vi "test.BasicTypes.vi"(8 "error in":errorcluster, 10 "Data":variant, 11 "Command":string) -> (0 "error out":errorcluster, 3 "Return Data":variant)   [LabVIEW 2014]
uses:
  Private/Class/class.GLue.lvclass
  Private/Class/meth.Constructor.vi
  Private/Class/meth.Destructor.vi
  GLue.lvlib
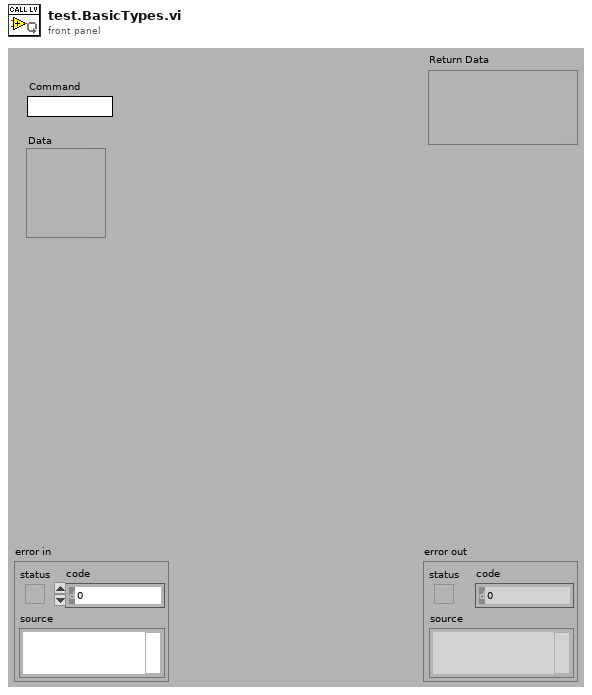
[diagram p1: front panel]
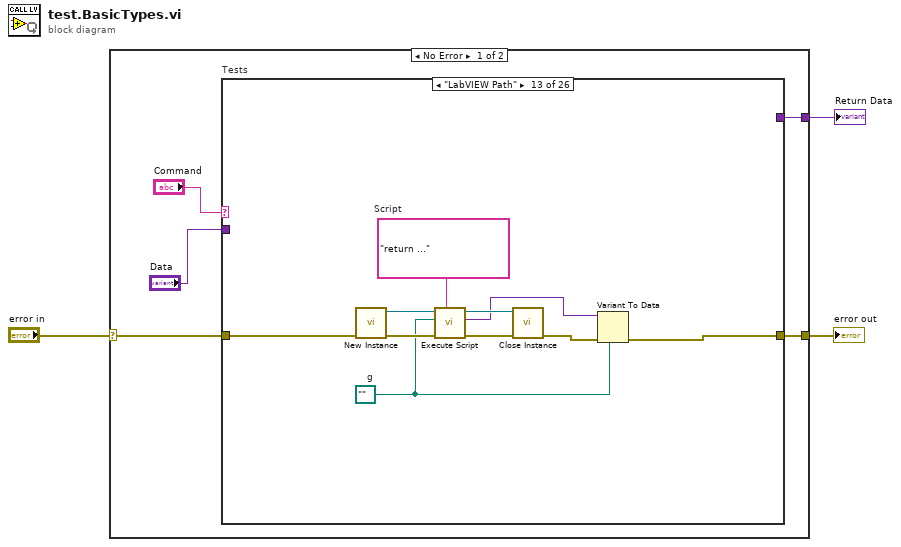
[diagram p0: block diagram]
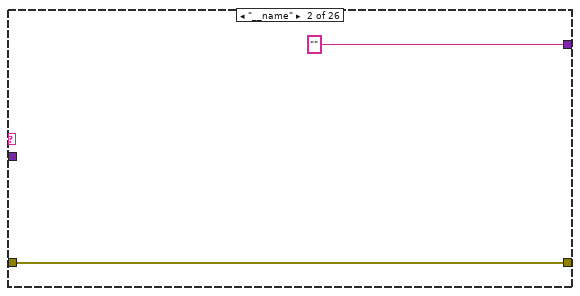
[diagram p3: hidden frame]
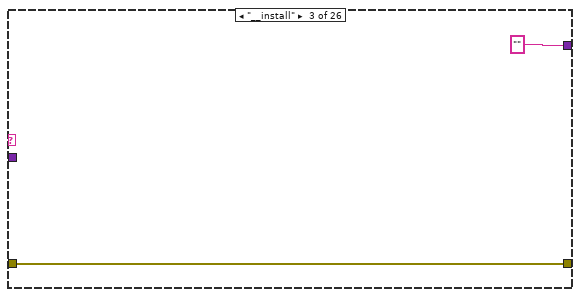
[diagram p4: hidden frame]
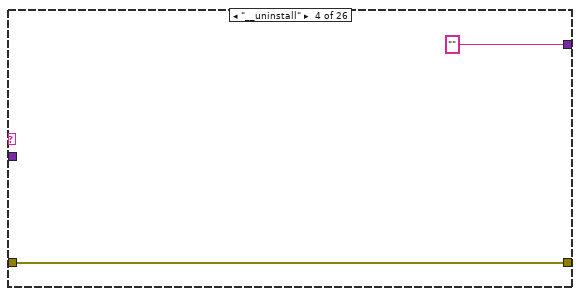
[diagram p5: hidden frame]
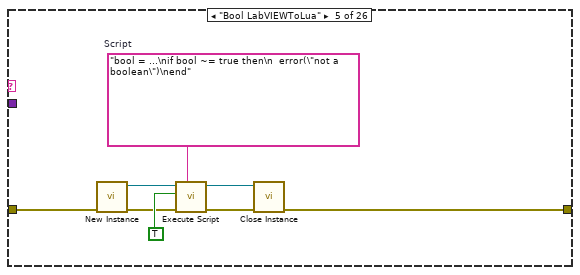
[diagram p6: hidden frame]
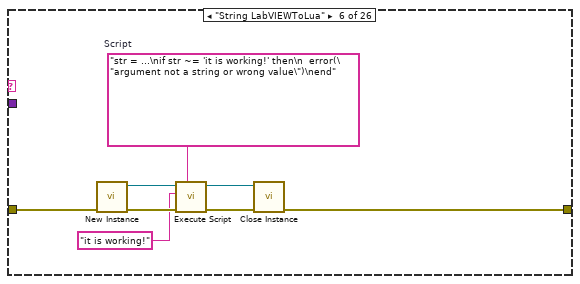
[diagram p7: hidden frame]
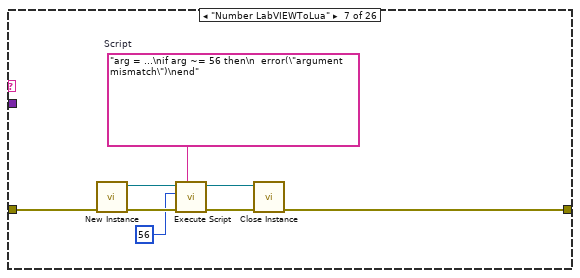
[diagram p8: hidden frame]
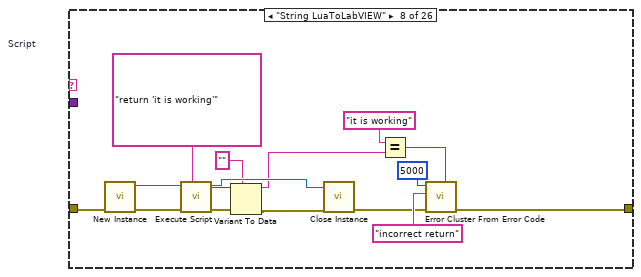
[diagram p9: hidden frame]
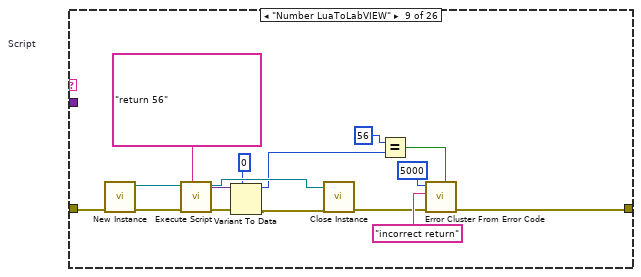
[diagram p10: hidden frame]
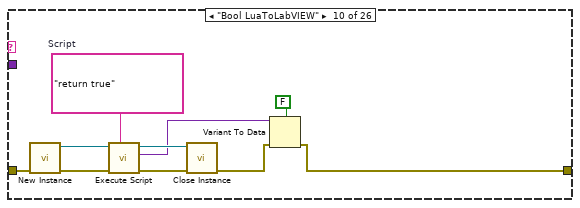
[diagram p11: hidden frame]
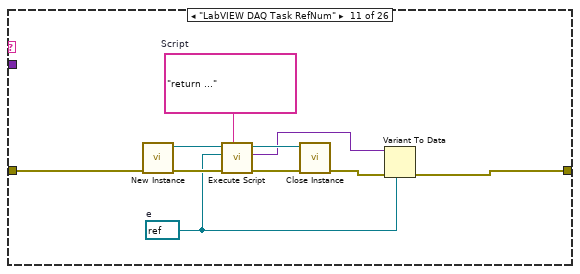
[diagram p12: hidden frame]
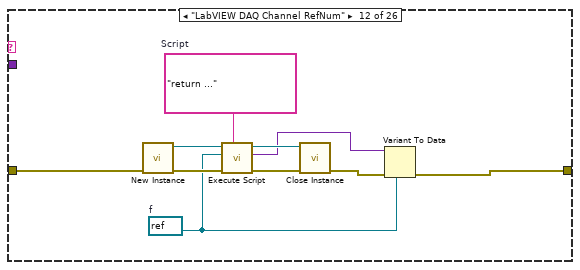
[diagram p13: hidden frame]
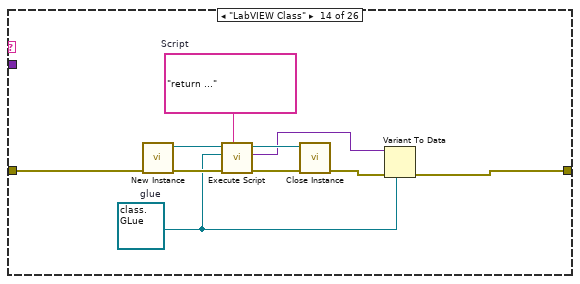
[diagram p14: hidden frame]
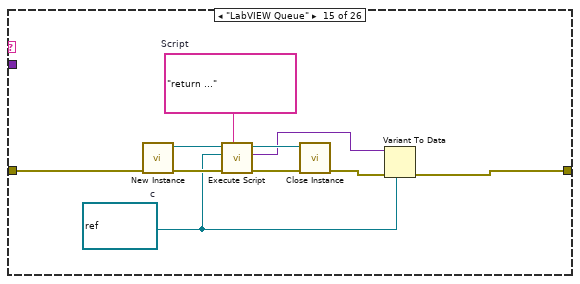
[diagram p15: hidden frame]
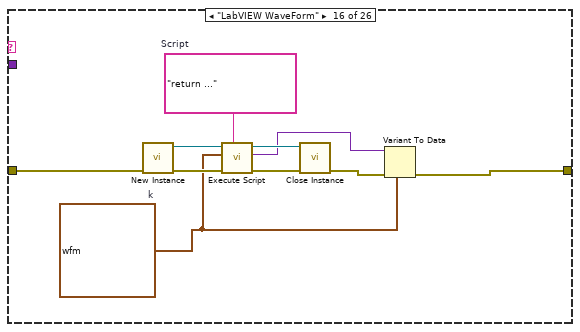
[diagram p16: hidden frame]
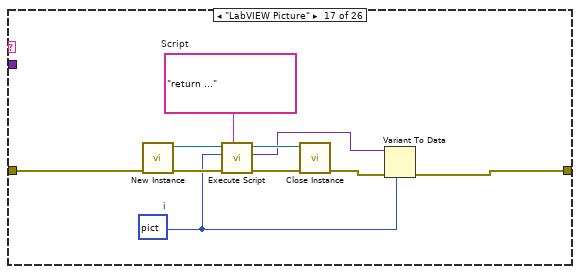
[diagram p17: hidden frame]
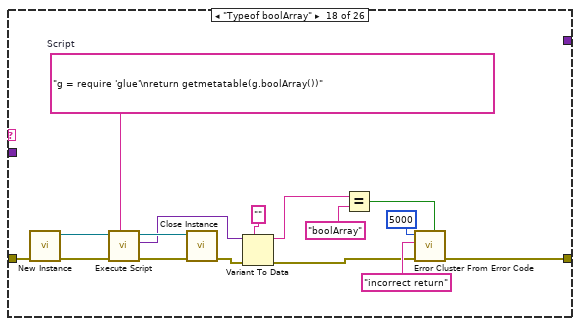
[diagram p18: hidden frame]
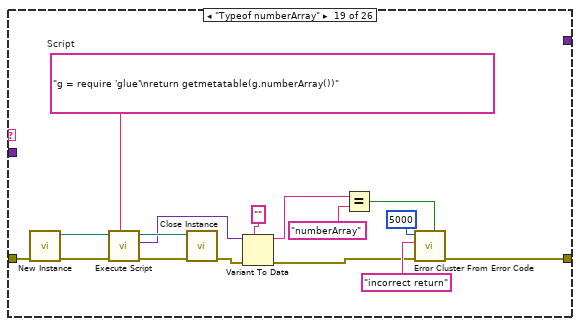
[diagram p19: hidden frame]
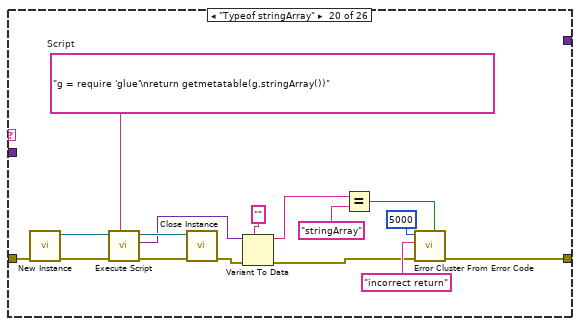
[diagram p20: hidden frame]
diagram:
  n1 = case shown="No Error" "error in" {
    selector: "error in" -> [w8 w297]
    tunnel: [w6 w297] -> w2
    tunnel: [w7 variant ("User Data")] -> w1
    frame No Error {
      n2 = case "Tests" shown="\"LabVIEW Path\"" "Command" {
        tunnel: w8 -> [w10 w11 w13 w15 w18 w27 w35 w53 w69 w77 w87 w97 w107 w117 w127 w137 w147 w163 w179 w195 w211 w227 w243 w260 w275 w290]
        tunnel: "Data" -> [w9 _ _ _ _ _ _ _ _ _ _ _ _ _ _ _ _ _ _ _ _ _ _ _ _ _]
        tunnel: [w9 "" "" "" _ _ _ _ _ _ _ _ _ _ _ _ _ _ _ _ _ _ _ _ _ _] -> w7
        tunnel: [w10 w11 w13 w15 w17 w26 w34 w41 w59 w73 w84 w94 w104 w114 w124 w134 w144 w156 w172 w188 w204 w220 w236 w253 w269 w284] -> w6
        frame Default {
        }
        frame "__name" {
        }
        frame "__install" {
        }
        frame "__uninstall" {
        }
        frame "Bool LabVIEWToLua" {
          w23 = "bool = ...\nif bool ~= true then\n  error(\"not a boolean\")\nend"  # Script
          n3 = call "New Instance.vi"("error in"=w18) -> ("error out"=w19:errorcluster, "GLue out"=w20:refnum<class "class.GLue.lvclass">)  [unwired: 9 in]
          n4 = call "Execute Script.vi"("Script"=w23, "error in"=w19, "Argument Data"=TRUE, "GLue in"=w20) -> ("error out"=w21:errorcluster, "GLue out"=w22:refnum<class "class.GLue.lvclass">)  [unwired: 5 in, 1 out]
          n5 = call "Close Instance.vi"("error in"=w21, "GLue in"=w22) -> ("error out"=w17:errorcluster)  [unwired: 9 in]
        }
        frame "String LabVIEWToLua" {
          w32 = "str = ...\nif str ~= 'it is working!' then\n  error(\"argument not a string or wrong value\")\nend"  # Script
          n6 = call "New Instance.vi"("error in"=w27) -> ("error out"=w28:errorcluster, "GLue out"=w29:refnum<class "class.GLue.lvclass">)  [unwired: 9 in]
          n7 = call "Execute Script.vi"("Script"=w32, "error in"=w28, "Argument Data"="it is working!", "GLue in"=w29) -> ("error out"=w30:errorcluster, "GLue out"=w31:refnum<class "class.GLue.lvclass">)  [unwired: 5 in, 1 out]
          n8 = call "Close Instance.vi"("error in"=w30, "GLue in"=w31) -> ("error out"=w26:errorcluster)  [unwired: 9 in]
        }
        frame "Number LabVIEWToLua" {
          w40 = "arg = ...\nif arg ~= 56 then\n  error(\"argument mismatch\")\nend"  # Script
          n9 = call "New Instance.vi"("error in"=w35) -> ("error out"=w36:errorcluster, "GLue out"=w37:refnum<class "class.GLue.lvclass">)  [unwired: 9 in]
          n10 = call "Execute Script.vi"("Script"=w40, "error in"=w36, "Argument Data"=56, "GLue in"=w37) -> ("error out"=w38:errorcluster, "GLue out"=w39:refnum<class "class.GLue.lvclass">)  [unwired: 5 in, 1 out]
          n11 = call "Close Instance.vi"("error in"=w38, "GLue in"=w39) -> ("error out"=w34:errorcluster)  [unwired: 9 in]
        }
        frame "String LuaToLabVIEW" {
          w56 = "return 'it is working'"  # Script
          n12 = call "New Instance.vi"("error in"=w53) -> ("error out"=w54:errorcluster, "GLue out"=w55:refnum<class "class.GLue.lvclass">)  [unwired: 9 in]
          n13 = call "Execute Script.vi"("Script"=w56, "error in"=w54, "GLue in"=w55) -> ("error out"=w52:errorcluster, "Return Data"=w51:variant, "GLue out"=w50:refnum<class "class.GLue.lvclass">)  [unwired: 6 in]
          n14 = Variant To Data(error in=w52, type="", Variant=w51) -> (data=w42:string, error out=w48:errorcluster)
          n15 = call "Close Instance.vi"("error in"=w48, "GLue in"=w50) -> ("error out"=w43:errorcluster)  [unwired: 9 in]
          n16 = Equal?(x="it is working" ("Function Name"), y=w42) -> (x = y?=w46:bool)
          n17 = call <vilib>:"Error Cluster From Error Code.vi"("is warning? (False)"=w46, "error in (no error)"=w43, "error message (\"\")"="incorrect return" ("error message (\"\")"), "error code (0)"=5000) -> ("error out"=w41:errorcluster)  [unwired: 5 in]
        }
        frame "Number LuaToLabVIEW" {
          w72 = "return 56"  # Script
          n18 = call "New Instance.vi"("error in"=w69) -> ("error out"=w70:errorcluster, "GLue out"=w71:refnum<class "class.GLue.lvclass">)  [unwired: 9 in]
          n19 = call "Execute Script.vi"("Script"=w72, "error in"=w70, "GLue in"=w71) -> ("error out"=w68:errorcluster, "Return Data"=w67:variant, "GLue out"=w66:refnum<class "class.GLue.lvclass">)  [unwired: 6 in]
          n20 = Variant To Data(error in=w68, type=0, Variant=w67) -> (data=w60:i32, error out=w65:errorcluster)
          n21 = call "Close Instance.vi"("error in"=w65, "GLue in"=w66) -> ("error out"=w61:errorcluster)  [unwired: 9 in]
          n22 = Equal?(x=56, y=w60) -> (x = y?=w64:bool)
          n23 = call <vilib>:"Error Cluster From Error Code.vi"("is warning? (False)"=w64, "error in (no error)"=w61, "error message (\"\")"="incorrect return" ("error message (\"\")"), "error code (0)"=5000) -> ("error out"=w59:errorcluster)  [unwired: 5 in]
        }
        frame "Bool LuaToLabVIEW" {
          w82 = "return true"  # Script
          n24 = call "New Instance.vi"("error in"=w77) -> ("error out"=w78:errorcluster, "GLue out"=w79:refnum<class "class.GLue.lvclass">)  [unwired: 9 in]
          n25 = call "Execute Script.vi"("Script"=w82, "error in"=w78, "GLue in"=w79) -> ("error out"=w80:errorcluster, "Return Data"=w75:variant, "GLue out"=w81:refnum<class "class.GLue.lvclass">)  [unwired: 6 in]
          n26 = call "Close Instance.vi"("error in"=w80, "GLue in"=w81) -> ("error out"=w74:errorcluster)  [unwired: 9 in]
          n27 = Variant To Data(error in=w74, type=FALSE, Variant=w75) -> (error out=w73:errorcluster)  [unwired: 1 out]
        }
        frame "LabVIEW DAQ Task RefNum" {
          w83 = refnum<k21> refnum  # e
          w92 = "return ..."  # Script
          n28 = call "New Instance.vi"("error in"=w87) -> ("error out"=w88:errorcluster, "GLue out"=w89:refnum<class "class.GLue.lvclass">)  [unwired: 9 in]
          n29 = call "Execute Script.vi"("Script"=w92, "error in"=w88, "Argument Data"=w83, "GLue in"=w89) -> ("error out"=w90:errorcluster, "Return Data"=w86:variant, "GLue out"=w91:refnum<class "class.GLue.lvclass">)  [unwired: 5 in]
          n30 = call "Close Instance.vi"("error in"=w90, "GLue in"=w91) -> ("error out"=w85:errorcluster)  [unwired: 9 in]
          n31 = Variant To Data(error in=w85, type=w83, Variant=w86) -> (error out=w84:errorcluster)  [unwired: 1 out]
        }
        frame "LabVIEW DAQ Channel RefNum" {
          w93 = refnum<k21> refnum  # f
          w102 = "return ..."  # Script
          n32 = call "New Instance.vi"("error in"=w97) -> ("error out"=w98:errorcluster, "GLue out"=w99:refnum<class "class.GLue.lvclass">)  [unwired: 9 in]
          n33 = call "Execute Script.vi"("Script"=w102, "error in"=w98, "Argument Data"=w93, "GLue in"=w99) -> ("error out"=w100:errorcluster, "Return Data"=w96:variant, "GLue out"=w101:refnum<class "class.GLue.lvclass">)  [unwired: 5 in]
          n34 = call "Close Instance.vi"("error in"=w100, "GLue in"=w101) -> ("error out"=w95:errorcluster)  [unwired: 9 in]
          n35 = Variant To Data(error in=w95, type=w93, Variant=w96) -> (error out=w94:errorcluster)  [unwired: 1 out]
        }
        frame "LabVIEW Path" {
          w103 = path ""  # g
          w112 = "return ..."  # Script
          n36 = call "New Instance.vi"("error in"=w107) -> ("error out"=w108:errorcluster, "GLue out"=w109:refnum<class "class.GLue.lvclass">)  [unwired: 9 in]
          n37 = call "Execute Script.vi"("Script"=w112, "error in"=w108, "Argument Data"=w103, "GLue in"=w109) -> ("error out"=w110:errorcluster, "Return Data"=w106:variant, "GLue out"=w111:refnum<class "class.GLue.lvclass">)  [unwired: 5 in]
          n38 = call "Close Instance.vi"("error in"=w110, "GLue in"=w111) -> ("error out"=w105:errorcluster)  [unwired: 9 in]
          n39 = Variant To Data(error in=w105, type=w103, Variant=w106) -> (error out=w104:errorcluster)  [unwired: 1 out]
        }
        frame "LabVIEW Class" {
          w113 = refnum<class "class.GLue.lvclass"> refnum  # glue
          w122 = "return ..."  # Script
          n40 = call "New Instance.vi"("error in"=w117) -> ("error out"=w118:errorcluster, "GLue out"=w119:refnum<class "class.GLue.lvclass">)  [unwired: 9 in]
          n41 = call "Execute Script.vi"("Script"=w122, "error in"=w118, "Argument Data"=w113, "GLue in"=w119) -> ("error out"=w120:errorcluster, "Return Data"=w116:variant, "GLue out"=w121:refnum<class "class.GLue.lvclass">)  [unwired: 5 in]
          n42 = call "Close Instance.vi"("error in"=w120, "GLue in"=w121) -> ("error out"=w115:errorcluster)  [unwired: 9 in]
          n43 = Variant To Data(error in=w115, type=w113, Variant=w116) -> (error out=w114:errorcluster)  [unwired: 1 out]
        }
        frame "LabVIEW Queue" {
          w123 = refnum<queue> refnum  # c
          w132 = "return ..."  # Script
          n44 = call "New Instance.vi"("error in"=w127) -> ("error out"=w128:errorcluster, "GLue out"=w129:refnum<class "class.GLue.lvclass">)  [unwired: 9 in]
          n45 = call "Execute Script.vi"("Script"=w132, "error in"=w128, "Argument Data"=w123, "GLue in"=w129) -> ("error out"=w130:errorcluster, "Return Data"=w126:variant, "GLue out"=w131:refnum<class "class.GLue.lvclass">)  [unwired: 5 in]
          n46 = call "Close Instance.vi"("error in"=w130, "GLue in"=w131) -> ("error out"=w125:errorcluster)  [unwired: 9 in]
          n47 = Variant To Data(error in=w125, type=w123, Variant=w126) -> (error out=w124:errorcluster)  [unwired: 1 out]
        }
        frame "LabVIEW WaveForm" {
          w133 = waveform(dbl) {"t0"=timestamp(0 s since 1904-01-01), "dt"=1.0, "Y"=[]}  # k
          w142 = "return ..."  # Script
          n48 = call "New Instance.vi"("error in"=w137) -> ("error out"=w138:errorcluster, "GLue out"=w139:refnum<class "class.GLue.lvclass">)  [unwired: 9 in]
          n49 = call "Execute Script.vi"("Script"=w142, "error in"=w138, "Argument Data"=w133, "GLue in"=w139) -> ("error out"=w140:errorcluster, "Return Data"=w136:variant, "GLue out"=w141:refnum<class "class.GLue.lvclass">)  [unwired: 5 in]
          n50 = call "Close Instance.vi"("error in"=w140, "GLue in"=w141) -> ("error out"=w135:errorcluster)  [unwired: 9 in]
          n51 = Variant To Data(error in=w135, type=w133, Variant=w136) -> (error out=w134:errorcluster)  [unwired: 1 out]
        }
        frame "LabVIEW Picture" {
          w143 = picture data[5B]  # i
          w152 = "return ..."  # Script
          n52 = call "New Instance.vi"("error in"=w147) -> ("error out"=w148:errorcluster, "GLue out"=w149:refnum<class "class.GLue.lvclass">)  [unwired: 9 in]
          n53 = call "Execute Script.vi"("Script"=w152, "error in"=w148, "Argument Data"=w143, "GLue in"=w149) -> ("error out"=w150:errorcluster, "Return Data"=w146:variant, "GLue out"=w151:refnum<class "class.GLue.lvclass">)  [unwired: 5 in]
          n54 = call "Close Instance.vi"("error in"=w150, "GLue in"=w151) -> ("error out"=w145:errorcluster)  [unwired: 9 in]
          n55 = Variant To Data(error in=w145, type=w143, Variant=w146) -> (error out=w144:errorcluster)  [unwired: 1 out]
        }
        frame "Typeof boolArray" {
          w168 = "g = require 'glue'\nreturn getmetatable(g.boolArray())"  # Script
          n56 = call "New Instance.vi"("error in"=w163) -> ("error out"=w164:errorcluster, "GLue out"=w165:refnum<class "class.GLue.lvclass">)  [unwired: 9 in]
          n57 = call "Execute Script.vi"("Script"=w168, "error in"=w164, "GLue in"=w165) -> ("error out"=w166:errorcluster, "Return Data"=w162:variant, "GLue out"=w167:refnum<class "class.GLue.lvclass">)  [unwired: 6 in]
          n58 = call "Close Instance.vi"("error in"=w166, "GLue in"=w167) -> ("error out"=w161:errorcluster)  [unwired: 9 in]
          n59 = Variant To Data(error in=w161, type="", Variant=w162) -> (data=w155:string, error out=w157:errorcluster)
          n60 = Equal?(x=w155, y="boolArray") -> (x = y?=w154:bool)
          n61 = call <vilib>:"Error Cluster From Error Code.vi"("is warning? (False)"=w154, "error in (no error)"=w157, "error message (\"\")"="incorrect return" ("error message (\"\")"), "error code (0)"=5000) -> ("error out"=w156:errorcluster)  [unwired: 5 in]
        }
        frame "Typeof numberArray" {
          w184 = "g = require 'glue'\nreturn getmetatable(g.numberArray())"  # Script
          n62 = call "New Instance.vi"("error in"=w179) -> ("error out"=w180:errorcluster, "GLue out"=w181:refnum<class "class.GLue.lvclass">)  [unwired: 9 in]
          n63 = call "Execute Script.vi"("Script"=w184, "error in"=w180, "GLue in"=w181) -> ("error out"=w182:errorcluster, "Return Data"=w178:variant, "GLue out"=w183:refnum<class "class.GLue.lvclass">)  [unwired: 6 in]
          n64 = call "Close Instance.vi"("error in"=w182, "GLue in"=w183) -> ("error out"=w177:errorcluster)  [unwired: 9 in]
          n65 = Variant To Data(error in=w177, type="", Variant=w178) -> (data=w171:string, error out=w173:errorcluster)
          n66 = Equal?(x=w171, y="numberArray") -> (x = y?=w170:bool)
          n67 = call <vilib>:"Error Cluster From Error Code.vi"("is warning? (False)"=w170, "error in (no error)"=w173, "error message (\"\")"="incorrect return" ("error message (\"\")"), "error code (0)"=5000) -> ("error out"=w172:errorcluster)  [unwired: 5 in]
        }
        frame "Typeof stringArray" {
          w200 = "g = require 'glue'\nreturn getmetatable(g.stringArray())"  # Script
          n68 = call "New Instance.vi"("error in"=w195) -> ("error out"=w196:errorcluster, "GLue out"=w197:refnum<class "class.GLue.lvclass">)  [unwired: 9 in]
          n69 = call "Execute Script.vi"("Script"=w200, "error in"=w196, "GLue in"=w197) -> ("error out"=w198:errorcluster, "Return Data"=w194:variant, "GLue out"=w199:refnum<class "class.GLue.lvclass">)  [unwired: 6 in]
          n70 = call "Close Instance.vi"("error in"=w198, "GLue in"=w199) -> ("error out"=w193:errorcluster)  [unwired: 9 in]
          n71 = Variant To Data(error in=w193, type="", Variant=w194) -> (data=w187:string, error out=w189:errorcluster)
          n72 = Equal?(x=w187, y="stringArray") -> (x = y?=w186:bool)
          n73 = call <vilib>:"Error Cluster From Error Code.vi"("is warning? (False)"=w186, "error in (no error)"=w189, "error message (\"\")"="incorrect return" ("error message (\"\")"), "error code (0)"=5000) -> ("error out"=w188:errorcluster)  [unwired: 5 in]
        }
        frame "Typeof clusterArray" {
          w216 = "g = require 'glue'\nreturn getmetatable(g.clusterArray())"  # Script
          n74 = call "New Instance.vi"("error in"=w211) -> ("error out"=w212:errorcluster, "GLue out"=w213:refnum<class "class.GLue.lvclass">)  [unwired: 9 in]
          n75 = call "Execute Script.vi"("Script"=w216, "error in"=w212, "GLue in"=w213) -> ("error out"=w214:errorcluster, "Return Data"=w210:variant, "GLue out"=w215:refnum<class "class.GLue.lvclass">)  [unwired: 6 in]
          n76 = call "Close Instance.vi"("error in"=w214, "GLue in"=w215) -> ("error out"=w209:errorcluster)  [unwired: 9 in]
          n77 = Variant To Data(error in=w209, type="", Variant=w210) -> (data=w203:string, error out=w205:errorcluster)
          n78 = Equal?(x=w203, y="clusterArray") -> (x = y?=w202:bool)
          n79 = call <vilib>:"Error Cluster From Error Code.vi"("is warning? (False)"=w202, "error in (no error)"=w205, "error message (\"\")"="incorrect return" ("error message (\"\")"), "error code (0)"=5000) -> ("error out"=w204:errorcluster)  [unwired: 5 in]
        }
        frame "Typeof cluster" {
          w232 = "g = require 'glue'\nreturn getmetatable(g.cluster())"  # Script
          n80 = call "New Instance.vi"("error in"=w227) -> ("error out"=w228:errorcluster, "GLue out"=w229:refnum<class "class.GLue.lvclass">)  [unwired: 9 in]
          n81 = call "Execute Script.vi"("Script"=w232, "error in"=w228, "GLue in"=w229) -> ("error out"=w230:errorcluster, "Return Data"=w226:variant, "GLue out"=w231:refnum<class "class.GLue.lvclass">)  [unwired: 6 in]
          n82 = call "Close Instance.vi"("error in"=w230, "GLue in"=w231) -> ("error out"=w225:errorcluster)  [unwired: 9 in]
          n83 = Variant To Data(error in=w225, type="", Variant=w226) -> (data=w219:string, error out=w221:errorcluster)
          n84 = Equal?(x=w219, y="cluster") -> (x = y?=w218:bool)
          n85 = call <vilib>:"Error Cluster From Error Code.vi"("is warning? (False)"=w218, "error in (no error)"=w221, "error message (\"\")"="incorrect return" ("error message (\"\")"), "error code (0)"=5000) -> ("error out"=w220:errorcluster)  [unwired: 5 in]
        }
        frame "Typeof variantWrapper" {
          w248 = "g = require 'glue'\nreturn getmetatable(g.toVariant('5'))"  # Script
          n86 = call "New Instance.vi"("error in"=w243) -> ("error out"=w244:errorcluster, "GLue out"=w245:refnum<class "class.GLue.lvclass">)  [unwired: 9 in]
          n87 = call "Execute Script.vi"("Script"=w248, "error in"=w244, "GLue in"=w245) -> ("error out"=w246:errorcluster, "Return Data"=w242:variant, "GLue out"=w247:refnum<class "class.GLue.lvclass">)  [unwired: 6 in]
          n88 = call "Close Instance.vi"("error in"=w246, "GLue in"=w247) -> ("error out"=w241:errorcluster)  [unwired: 9 in]
          n89 = Variant To Data(error in=w241, type="", Variant=w242) -> (data=w235:string, error out=w237:errorcluster)
          n90 = Equal?(x=w235, y="variantWrapper") -> (x = y?=w234:bool)
          n91 = call <vilib>:"Error Cluster From Error Code.vi"("is warning? (False)"=w234, "error in (no error)"=w237, "error message (\"\")"="incorrect return" ("error message (\"\")"), "error code (0)"=5000) -> ("error out"=w236:errorcluster)  [unwired: 5 in]
        }
        frame "Typeof variant" {
          w265 = "g = require 'glue'\nreturn getmetatable(...)"  # Script
          n92 = call "New Instance.vi"("error in"=w260) -> ("error out"=w261:errorcluster, "GLue out"=w262:refnum<class "class.GLue.lvclass">)  [unwired: 9 in]
          n93 = control-ref of="This VI"() -> (w249:refnum<vi>)
          n94 = call "Execute Script.vi"("Script"=w265, "error in"=w261, "Argument Data"=w249, "GLue in"=w262) -> ("error out"=w263:errorcluster, "Return Data"=w259:variant, "GLue out"=w264:refnum<class "class.GLue.lvclass">)  [unwired: 5 in]
          n95 = call "Close Instance.vi"("error in"=w263, "GLue in"=w264) -> ("error out"=w258:errorcluster)  [unwired: 9 in]
          n96 = Variant To Data(error in=w258, type="", Variant=w259) -> (data=w252:string, error out=w254:errorcluster)
          n97 = Equal?(x=w252, y="variant") -> (x = y?=w251:bool)
          n98 = call <vilib>:"Error Cluster From Error Code.vi"("is warning? (False)"=w251, "error in (no error)"=w254, "error message (\"\")"="incorrect return" ("error message (\"\")"), "error code (0)"=5000) -> ("error out"=w253:errorcluster)  [unwired: 5 in]
        }
        frame "Glue Not Loaded By Default" {
          w280 = "return glue == nil"  # Script
          n99 = call "New Instance.vi"("error in"=w275) -> ("error out"=w276:errorcluster, "GLue out"=w277:refnum<class "class.GLue.lvclass">)  [unwired: 9 in]
          n100 = control-ref of="This VI"() -> (w268:refnum<vi>)
          n101 = call "Execute Script.vi"("Script"=w280, "error in"=w276, "Argument Data"=w268, "GLue in"=w277) -> ("error out"=w278:errorcluster, "Return Data"=w274:variant, "GLue out"=w279:refnum<class "class.GLue.lvclass">)  [unwired: 5 in]
          n102 = call "Close Instance.vi"("error in"=w278, "GLue in"=w279) -> ("error out"=w273:errorcluster)  [unwired: 9 in]
          n103 = Variant To Data(error in=w273, type=TRUE, Variant=w274) -> (data=w266:bool, error out=w270:errorcluster)
          n104 = call <vilib>:"Error Cluster From Error Code.vi"("is warning? (False)"=w266, "error in (no error)"=w270, "error message (\"\")"="incorrect return" ("error message (\"\")"), "error code (0)"=5000) -> ("error out"=w269:errorcluster)  [unwired: 5 in]
        }
        frame "Glue Loaded By Require" {
          w295 = "glue = require 'glue'\nreturn glue ~= nil"  # Script
          n105 = call "New Instance.vi"("error in"=w290) -> ("error out"=w291:errorcluster, "GLue out"=w292:refnum<class "class.GLue.lvclass">)  [unwired: 9 in]
          n106 = control-ref of="This VI"() -> (w283:refnum<vi>)
          n107 = call "Execute Script.vi"("Script"=w295, "error in"=w291, "Argument Data"=w283, "GLue in"=w292) -> ("error out"=w293:errorcluster, "Return Data"=w289:variant, "GLue out"=w294:refnum<class "class.GLue.lvclass">)  [unwired: 5 in]
          n108 = call "Close Instance.vi"("error in"=w293, "GLue in"=w294) -> ("error out"=w288:errorcluster)  [unwired: 9 in]
          n109 = Variant To Data(error in=w288, type=TRUE, Variant=w289) -> (data=w281:bool, error out=w285:errorcluster)
          n110 = call <vilib>:"Error Cluster From Error Code.vi"("is warning? (False)"=w281, "error in (no error)"=w285, "error message (\"\")"="incorrect return" ("error message (\"\")"), "error code (0)"=5000) -> ("error out"=w284:errorcluster)  [unwired: 5 in]
        }
      }
    }
    frame Error {
    }
  }
  "Return Data" <- w1
  "error out" <- w2
